vi "LEDeezNuts Loop.vi"   [LabVIEW 2016]
uses:
  <vilib>/Rock Robotics/WPI/DriverStation/WPI_DriverStationRobotMode2.ctl
  Common Code/LED Indicator.ctl
  Robot Global Data.vi
  <vilib>/Rock Robotics/WPI/Solenoid/Deprecated/WPI_SolenoidSetBool.vi
types:
  T1 = typedef "WPI_DriverStationRobotMode2.ctl" = enum16{"Autonomous Disabled", "Autonomous Enabled", "Teleop Disabled", "Teleop Enabled", "Disconnected", "Finish", "Test Disabled", "Test Enabled", "Emergency Stopped"}
  T2 = typedef "Intake Control Cluster.ctl" = cluster{"Intake Mode":T3, "Intake Auto Command":T4, "Intake Current Trip State":T5, "Gear slot open?":bool, "Engage traction for gear load?":bool, "Wings open?":bool, "Manual Intake Power":dbl}
  T3 = typedef "Intake Modes.ctl" = enum16{"Manual", "Auto"}
  T4 = typedef "Intake Auto States.ctl" = enum16{"Outake Ball", "Idle", "Load Ball"}
  T5 = typedef "Intake Trip States.ctl" = enum16{"Normal", "Backward Tripped", "Forward Tripped"}
  T6 = typedef "Drivetrain Command Cluster.ctl" = cluster{"Drivetrain Mode":T7, "Heading Target":dbl, "Turn Power":dbl, "Y Power":dbl, "Center Piston Down?":bool, "Traction?":bool, "Strafe Power":dbl, "Zero Gyro":bool, "Distance Target":dbl, "Strafe Correct":bool, "Y Max Output":dbl, "Y Min Output":dbl, "X Max Output":dbl, "X Min Output":dbl, "Z Max Output":dbl, "Z Min Output":dbl, "Z Target":dbl, "Brake?":bool}
  T7 = typedef "Drivetrain Mode.ctl" = enum16{"Manual", "Gyro Steer", "Distance Drive", "Translate Drive", "Goal Vision Align", "PID Drive"}
  T8 = typedef "LED Indicator.ctl" = enum16{"BrakeOn", "GearReady", "Traction", "Intake", "None"}
  T9 = typedef "WPI_SolenoidDevRef.ctl" = cluster{"DevStatus":errorcluster, "Pneumatics Control Module":u8, "Forward Solenoid Channel":T10, "Reverse Solenoid Channel":T10}
  T10 = typedef "WPI_SolenoidChannel.ctl" = enum8{"Solenoid 0", "Solenoid 1", "Solenoid 2", "Solenoid 3", "Solenoid 4", "Solenoid 5", "Solenoid 6", "Solenoid 7", "Invalid"}
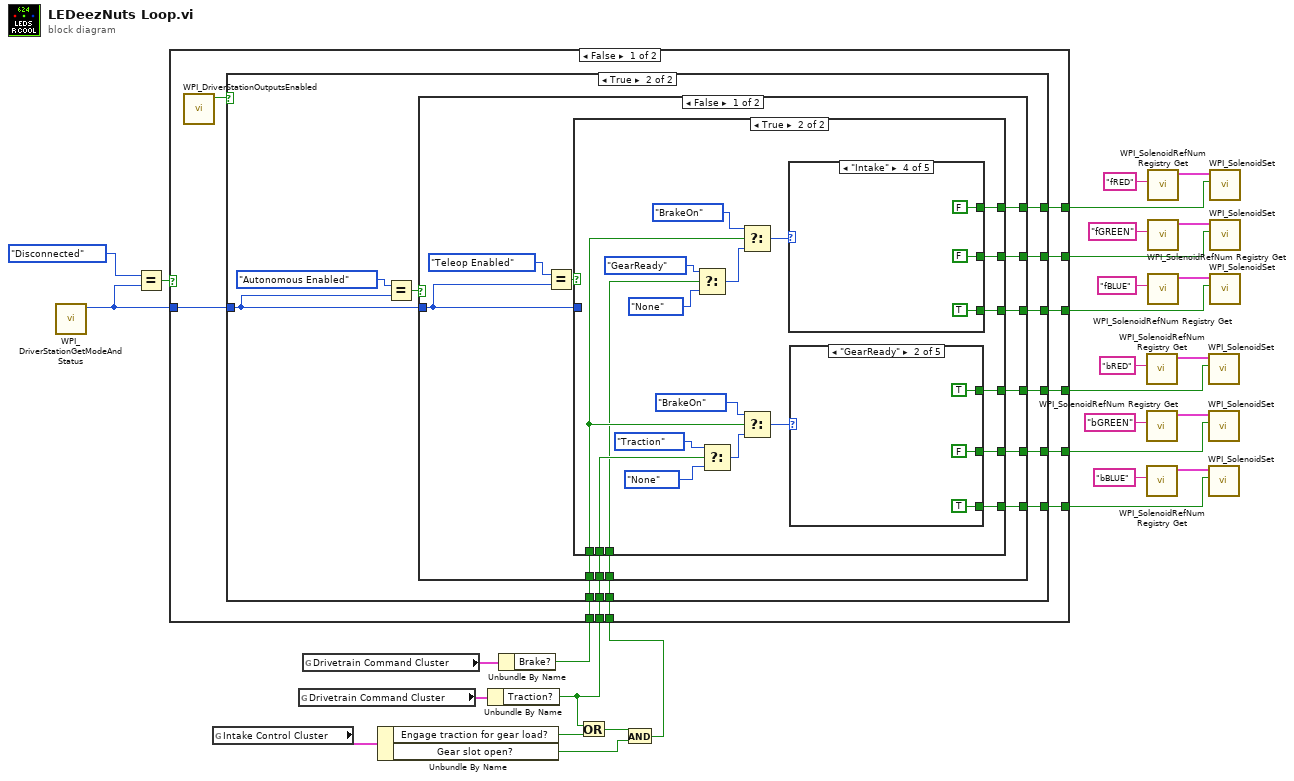
[diagram p0: block diagram]
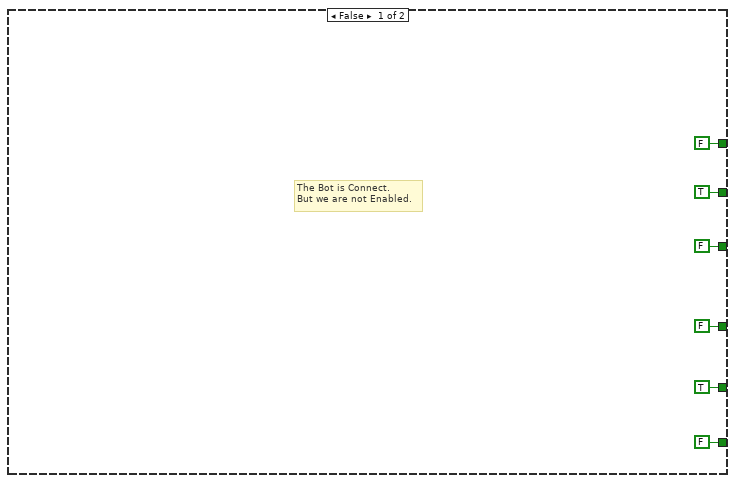
[diagram p2: hidden frame]
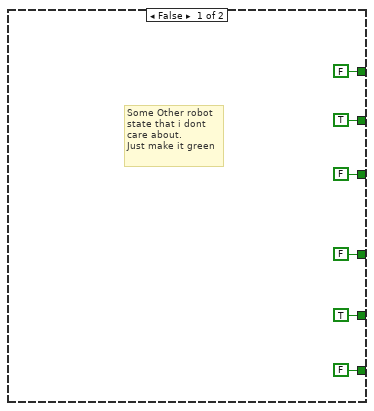
[diagram p3: hidden frame]
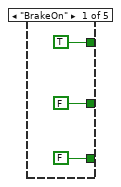
[diagram p4: hidden frame]
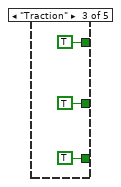
[diagram p5: hidden frame]
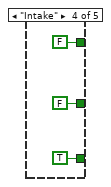
[diagram p6: hidden frame]
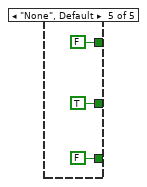
[diagram p7: hidden frame]
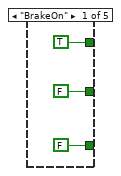
[diagram p8: hidden frame]
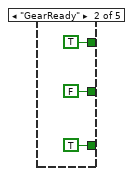
[diagram p9: hidden frame]
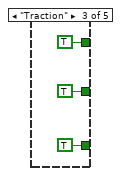
[diagram p10: hidden frame]
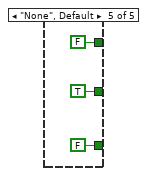
[diagram p11: hidden frame]
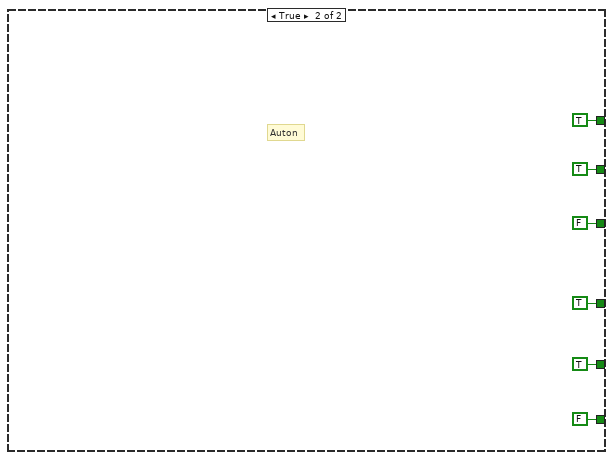
[diagram p12: hidden frame]
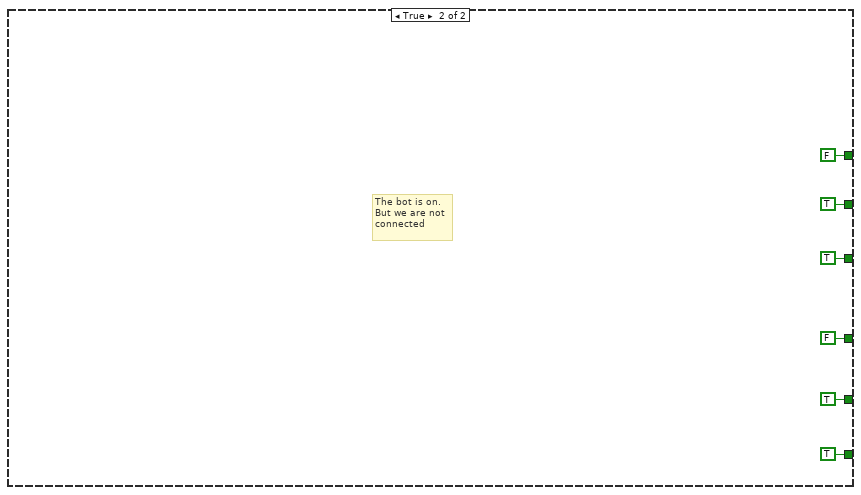
[diagram p13: hidden frame]
diagram:
  n1 = call <vilib>:"WPI_DriverStationGetModeAndStatus.vi"() -> ("Robot Mode"=w23:T1)  [unwired: 10 in, 1 out]
  n2 = Equal?(x=WPI_DriverStationRobotMode2."Disconnected" ("Robot Mode"), y=w23) -> (x = y?=w24:bool)
  n3 = global read "Robot Global Data.vi" "Intake Control Cluster"() -> (w12:T2)
  n4 = global read "Robot Global Data.vi" "Drivetrain Command Cluster"() -> (w21:T6)
  n5 = global read "Robot Global Data.vi" "Drivetrain Command Cluster"() -> (w14:T6)
  n6 = Unbundle By Name(w12) -> ("Engage traction for gear load?"=w5:bool, "Gear slot open?"=w2:bool)
  n7 = Unbundle By Name(w21) -> ("Traction?"=w4:bool)
  n8 = Unbundle By Name(w14) -> ("Brake?"=w13:bool)
  n9 = Or(x=w4, y=w5) -> (x .or. y?=w3:bool)
  n10 = And(x=w3, y=w2) -> (x .and. y?=w1:bool)
  n11 = case shown="False" w24 {
    tunnel: w23 -> [w40 _]
    tunnel: w4 -> [w39 _]
    tunnel: w13 -> [w38 _]
    tunnel: w1 -> [w37 _]
    tunnel: [w36 TRUE] -> w11
    tunnel: [w35 TRUE] -> w10
    tunnel: [w34 FALSE] -> w9
    tunnel: [w33 TRUE] -> w8
    tunnel: [w32 TRUE] -> w7
    tunnel: [w31 FALSE] -> w6
    frame False {
      n12 = call <vilib>:"WPI_DriverStationOutputsEnabled.vi"() -> ("OutputsEnabled?"=w41:bool)  [unwired: 10 in, 1 out]
      n13 = case shown="True" w41 {
        tunnel: w40 -> [_ w57]
        tunnel: w39 -> [_ w56]
        tunnel: w38 -> [_ w55]
        tunnel: w37 -> [_ w54]
        tunnel: [FALSE w53] -> w36
        tunnel: [TRUE w52] -> w35
        tunnel: [FALSE w51] -> w34
        tunnel: [FALSE w50] -> w33
        tunnel: [TRUE w49] -> w32
        tunnel: [FALSE w48] -> w31
        frame False {
          # "The Bot is Connect.\nBut we are not Enabled."
        }
        frame True {
          n14 = Equal?(x=WPI_DriverStationRobotMode2."Autonomous Enabled" ("Robot Mode"), y=w57) -> (x = y?=w58:bool)
          n15 = case shown="False" w58 {
            tunnel: w57 -> [w69 _]
            tunnel: w56 -> [w68 _]
            tunnel: w55 -> [w67 _]
            tunnel: w54 -> [w66 _]
            tunnel: [w65 FALSE] -> w53
            tunnel: [w64 TRUE] -> w52
            tunnel: [w63 TRUE] -> w51
            tunnel: [w62 FALSE] -> w50
            tunnel: [w61 TRUE] -> w49
            tunnel: [w60 TRUE] -> w48
            frame False {
              n16 = Equal?(x=WPI_DriverStationRobotMode2."Teleop Enabled" ("Robot Mode"), y=w69) -> (x = y?=w70:bool)
              n17 = case shown="True" w70 {
                tunnel: w69 -> [_ _]
                tunnel: w68 -> [_ w94]
                tunnel: w67 -> [_ w93]
                tunnel: w66 -> [_ w85]
                tunnel: [FALSE w83] -> w65
                tunnel: [TRUE w82] -> w64
                tunnel: [FALSE w81] -> w63
                tunnel: [FALSE w80] -> w62
                tunnel: [TRUE w79] -> w61
                tunnel: [FALSE w78] -> w60
                frame False {
                  # "Some Other robot\nstate that i dont\ncare about.\nJust make it green"
                }
                frame True {
                  n18 = Select(t=LED_Indicator."GearReady" ("Enum"), s=w85, f=LED_Indicator."None" ("Enum")) -> (s? t:f=w91:T8)
                  n19 = Select(t=LED_Indicator."Traction" ("Enum"), s=w94, f=LED_Indicator."None" ("Enum")) -> (s? t:f=w95:T8)
                  n20 = Select(t=LED_Indicator."BrakeOn" ("Enum"), s=w93, f=w91) -> (s? t:f=w88:T8)
                  n21 = Select(t=LED_Indicator."BrakeOn" ("Enum"), s=w93, f=w95) -> (s? t:f=w89:T8)
                  n22 = case shown="\"Intake\"" w88 {
                    tunnel: [FALSE TRUE TRUE TRUE FALSE] -> w83
                    tunnel: [FALSE FALSE TRUE FALSE TRUE] -> w82
                    tunnel: [TRUE TRUE TRUE FALSE FALSE] -> w81
                    frame "BrakeOn" {
                    }
                    frame "GearReady" {
                    }
                    frame "Traction" {
                    }
                    frame "Intake" {
                    }
                    frame "None", Default {
                    }
                  }
                  n23 = case shown="\"GearReady\"" w89 {
                    tunnel: [FALSE TRUE TRUE TRUE FALSE] -> w80
                    tunnel: [FALSE FALSE TRUE FALSE TRUE] -> w79
                    tunnel: [TRUE TRUE TRUE FALSE FALSE] -> w78
                    frame "BrakeOn" {
                    }
                    frame "GearReady" {
                    }
                    frame "Traction" {
                    }
                    frame "Intake" {
                    }
                    frame "None", Default {
                    }
                  }
                }
              }
            }
            frame True {
              # "Auton"
            }
          }
        }
      }
    }
    frame True {
      # "The bot is on.\nBut we are not\nconnected"
    }
  }
  n24 = call <vilib>:"WPI_SolenoidRefNum Registry Get.vi"("refnum name"="bRED") -> ("SolenoidDevRef"=w15:T9)  [unwired: 9 in, 1 out]
  n25 = call <vilib>:"WPI_SolenoidRefNum Registry Get.vi"("refnum name"="bGREEN") -> ("SolenoidDevRef"=w18:T9)  [unwired: 9 in, 1 out]
  n26 = call <vilib>:"WPI_SolenoidRefNum Registry Get.vi"("refnum name"="bBLUE") -> ("SolenoidDevRef"=w19:T9)  [unwired: 9 in, 1 out]
  n27 = call <vilib>:"WPI_SolenoidRefNum Registry Get.vi"("refnum name"="fRED") -> ("SolenoidDevRef"=w30:T9)  [unwired: 9 in, 1 out]
  n28 = call <vilib>:"WPI_SolenoidRefNum Registry Get.vi"("refnum name"="fGREEN") -> ("SolenoidDevRef"=w27:T9)  [unwired: 9 in, 1 out]
  n29 = call <vilib>:"WPI_SolenoidRefNum Registry Get.vi"("refnum name"="fBLUE") -> ("SolenoidDevRef"=w26:T9)  [unwired: 9 in, 1 out]
  n30 = call-poly <vilib>:"WPI_SolenoidSet.vi"("Value"=w6, "SolenoidDevRef"=w15) -> ()  [unwired: 8 in, 2 out]
  n31 = call-poly <vilib>:"WPI_SolenoidSet.vi"("Value"=w7, "SolenoidDevRef"=w18) -> ()  [unwired: 8 in, 2 out]
  n32 = call-poly <vilib>:"WPI_SolenoidSet.vi"("Value"=w8, "SolenoidDevRef"=w19) -> ()  [unwired: 8 in, 2 out]
  n33 = call-poly <vilib>:"WPI_SolenoidSet.vi"("Value"=w9, "SolenoidDevRef"=w30) -> ()  [unwired: 8 in, 2 out]
  n34 = call-poly <vilib>:"WPI_SolenoidSet.vi"("Value"=w10, "SolenoidDevRef"=w27) -> ()  [unwired: 8 in, 2 out]
  n35 = call-poly <vilib>:"WPI_SolenoidSet.vi"("Value"=w11, "SolenoidDevRef"=w26) -> ()  [unwired: 8 in, 2 out]
